vi "Test_RetrieveNextItem_RetrieveItem.vi"(8 "error in (no error)":errorcluster, 11 "TestCase in":refnum<class "TestStringList.lvclass">) -> (0 "error out":errorcluster, 3 "TestCase out":refnum<class "TestStringList.lvclass">)   [LabVIEW 2015, in "StringList.lvlib" / "TestStringList.lvclass"]
uses:
  TestStringList.lvclass
  <vilib>/addons/_JKI Toolkits/VI Tester/TestCase.llb/TestCase.lvclass
  StringList.lvclass
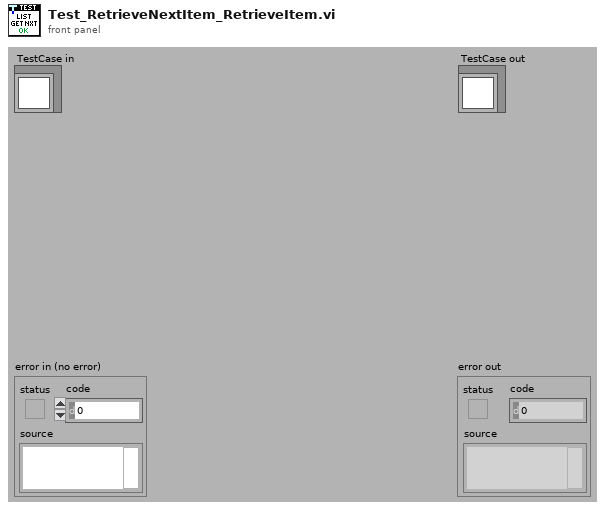
[diagram p1: front panel]
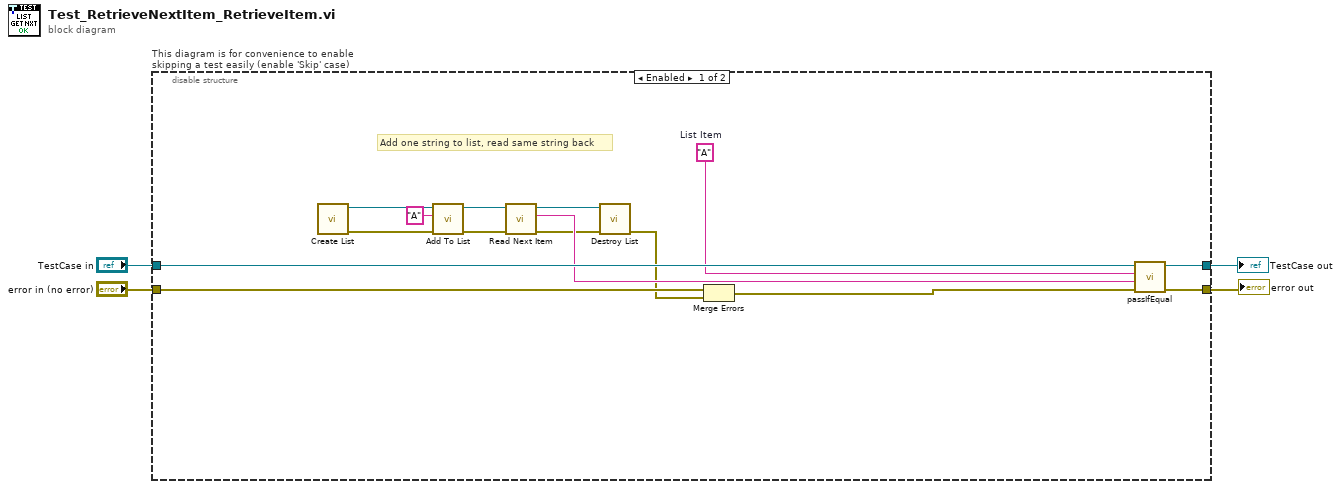
[diagram p0: block diagram]
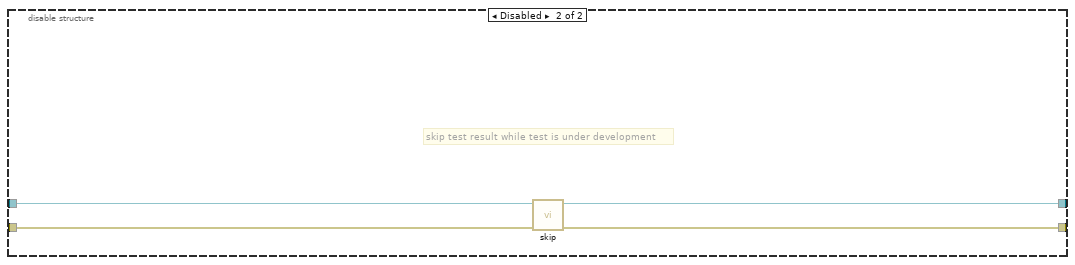
[diagram p2: hidden frame]
diagram:
  n1 = disable-structure "This diagram is for convenience to enable skipping a test easily (enable 'Skip' case)" shown="Enabled" {
    disable-tunnel: "TestCase in" -> [w19 w23]
    disable-tunnel: [w18 w21] -> w1
    disable-tunnel: [w17 w22] -> w3
    disable-tunnel: "error in (no error)" -> [w16 w20]
    frame Enabled {
      w14 = "A"  # List Item
      # "Add one string to list, read same string back"
      n2 = call "Create List.vi"() -> ("error out"=w9:errorcluster, "StringList Reference"=w11:refnum<data-value>)  [unwired: 10 in]
      n3 = call "Add To List.vi"("error in (no error)"=w9, "Item"="A" ("String"), "StringList Reference"=w11) -> ("error out"=w8:errorcluster, "StringList Reference"=w13:refnum<data-value>)  [unwired: 7 in]
      n4 = call "Read Next Item.vi"("error in (no error)"=w8, "StringList Reference"=w13) -> ("error out"=w7:errorcluster, "Item"=w15:string, "StringList Reference"=w10:refnum<data-value>)  [unwired: 6 in, 1 out]
      n5 = call "Destroy List.vi"("error in (no error)"=w7, "StringList Reference"=w10) -> ("error out"=w5:errorcluster)  [unwired: 8 in, 1 out]
      n6 = Merge Errors(w16, w5) -> (w6:errorcluster)
      n7 = call-dynamic "passIfEqual.vi"("error in (no error)"=w6, "y"=w15, "x"=w14, "TestCase in"=w19) -> ("error out"=w17:errorcluster, "TestCase out"=w18:refnum<class "TestStringList.lvclass">)  [unwired: 6 in]
    }
    frame Disabled {
      # "skip test result while test is under development"
      n8 = call <vilib>:"skip.vi"("error in (no error)"=w20, "TestCase in"=w23) -> ("error out"=w22:errorcluster, "TestCase out"=w21:refnum<class "TestStringList.lvclass">)  [unwired: 8 in]
    }
  }
  "error out" <- w3
  "TestCase out" <- w1
